vi "Dashboard Main.vi"() -> ()   [LabVIEW 2013]
uses:
  <vilib>/event_ctls.llb/eventvkey.ctl
  <vilib>/Rock Robotics/WPI/Dashboard/WPI_DashboardLogging Global.vi
  <vilib>/Utility/config.llb/Write Key (String).vi
  <vilib>/Utility/config.llb/Write Key (I32).vi
  <vilib>/Utility/config.llb/NI_LVConfig.lvlib
panel:
  out "Image Message":string="Timeout in Camera Communications"
  in  "Rec Mode":enum32{"Stop", "Record", "Playback"}(radio)
  in  "Dashboard Tab":T1(tab)
  in  "Camera Settings":T2={"Frame Rate"=30, "Compression"=30, "Size"=1} {"Frame Rate" scale=1.0..30.0; "Size" items=["640x480", "320x240", "160x120"]}
  out "MotorSliders R":T3 {"MotorSlide2 2" scale=-1.0..1.0 scale format="%#_2e"; "MotorSlide2" scale=-1.0..1.0 scale format="%#_2e"; "MotorSlide1" scale=-1.0..1.0 scale format="%#_2e"}
  out "MotorSliders L":T4 {"MotorSlide2" scale=-1.0..1.0 scale format="%#_2e"; "MotorSlide2 2" scale=-1.0..1.0 scale format="%#_2e"; "MotorSlide4 2" scale=0.0..14.0 scale format="%#_2e"; "MotorSlide1" scale=-1.0..1.0 scale format="%#_2e"}
  out "MotorChart L":T5(graph)
  out "JS1 Z":dbl(slide) scale=-1.0..1.0 scale format="%#_2e"
  out "L Joystick":cluster{"X":dbl, "Y":dbl}[](graph)
  out "JS Buttons 1":T6
  out "JS2 Z":dbl(slide) scale=-1.0..1.0 scale format="%#_2e"
  out "R Joystick":cluster{"X":dbl, "Y":dbl}[](graph)
  out "JS Buttons 2":T6
  out "Mode":T7(ring)=enum."Auto Disabled"
  out "Camera IP":string
  in  "DB Camera Config":bool
  out "fps":dbl format="%#.1g"
  out "Mbps":dbl format="%#.1g"
  out "Mbps 2":bool
  out "Target Cnt (RPi)":dbl
  out "Target Cnt (RIO)":dbl
  out "MotorChart R":T8(graph)
  in  "Enable Vision":bool
  in  "Slider 1":dbl(slide) scale=0.0..100.0
  in  "Checkbox 2":bool
  in  "Checkbox 1":bool
  in  "Test Slider":dbl(slide) scale=0.0..100.0 scale format="%#_3g"
  in  "On/Off":bool caption="Solenoid"
  in  "Test Name":u16(ring) items=["Select the test to run...", "Example Test", "-------------------------------", "List of tests is built in robot code.", "Replace with your own automated tests."]
  in  "Test Tree":string(tree)
  in  "Motor":cluster{"Value":dbl, "Enable":bool} {"Value" scale=-1.0..1.0 scale format="%#_3g"}
  out "Progress":T9 {"Test Progress" scale=0.0..100.0}
  in  "Rev/Fwd":cluster{"Forward":bool, "Reverse":bool}
  in  "Test Ring":u16(ring) items=["Auto", "Fixed indoor", "Fixed outdoor 1", "Fixed outdoor 2", "Fixed fluorescent 1", "Fixed fluorescent 2", "Hold current"]
  in  "Listbox":i32(listbox)
  out "Tree":string(tree)
  out "Camera Image":T10(plugin-control)
  in  "Enable":bool
  # "Left"
  # "Front"
  # "Right"
  # "Battery"
  # "Customize by placing controls and indicators here and name to\nmatch Dashboard Variables on robot."
  # "This tab is a great place for autonomous settings and validation.\nCustomize by placing controls and indicators here and name to\nmatch Dashboard Variables on robot."
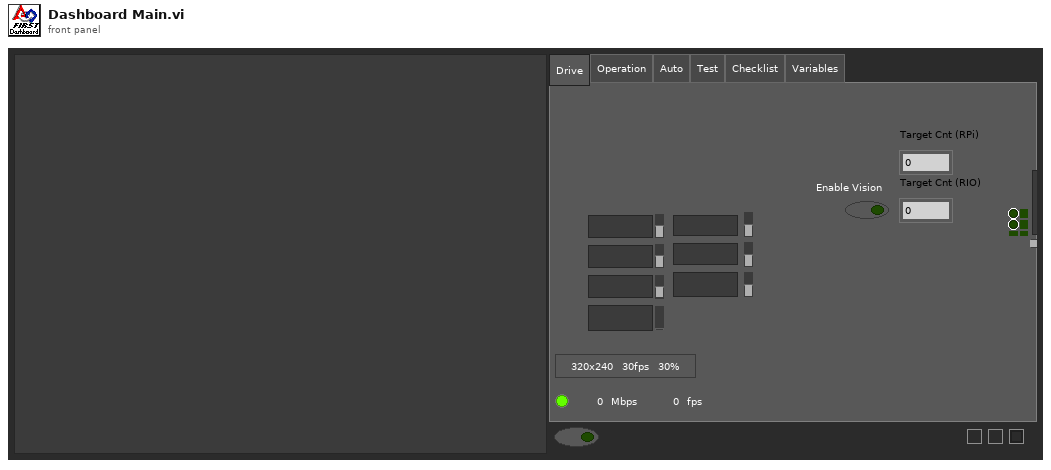
[diagram p1: front panel]
types:
  T1 = enum32{"Drive", "Operation", "Auto", "Test", "Checklist", "Variables"}
  T2 = cluster{"Frame Rate":i32, "Compression":i32, "Size":u16}
  T3 = cluster{"MotorSlide1":dbl, "MotorSlide2":dbl, "MotorSlide2 2":dbl}
  T4 = cluster{"MotorSlide1":dbl, "MotorSlide4 2":dbl, "MotorSlide2 2":dbl, "MotorSlide2":dbl}
  T5 = cluster{"Numeric":dbl, "Numeric":dbl, "Numeric":dbl, "Battery":sgl}
  T6 = cluster{bool, bool, bool, bool, bool, bool, bool, bool, bool, bool, bool, bool}
  T7 = enum8{"Tele-Op Disabled", "Tele-Op Enabled", "Auto Disabled", "Auto Enabled", "Test Disabled", "Test Enabled", ""}
  T8 = cluster{"Numeric":dbl, "Numeric":dbl, "Numeric":dbl}
  T9 = cluster{"Test Progress":u8, "Test Progress Text":string}
  T10 = typedef "IMAQ Image.ctl" = refnum<image>
  T11 = typedef "Image Type" = u32
  T12 = cluster{"Digital Inputs":bool[], "Digital Outputs":bool[]}
  T13 = cluster{"Competition mode":bool, "Robot Link":bool, "Autonomous":bool, "Enabled":bool, "E-Stop":bool, "Simulated":bool, "TestMode":bool, "Docked Window":bool}
  T14 = cluster{"Boolean Array[0]":bool, "Boolean Array[1]":bool, "Boolean Array[2]":bool, "Boolean Array[3]":bool, "Boolean Array[4]":bool, "Boolean Array[5]":bool, "Boolean Array[6]":bool, "Boolean Array[7]":bool, "Boolean Array[8]":bool, "Boolean Array[9]":bool, "Boolean Array[10]":bool, "Boolean Array[11]":bool}
  T15 = typedef "NI_LVConfig.lvlib/Config Data RefNum.ctl" = refnum<k1>
  T16 = typedef "eventvkey.ctl" = enum16{"ASCII", "Enter", "Return", "Shift", "Ctrl", "Alt", "Cmd", "Opt", "Caps", "NumLock", "Clear", "Break", "Up", "Down", "Left", "Right", "Insert", "Delete", "Home", "End", "PageUp", "PageDown", "Escape", "Help", "Pause", "ScrollLock", "F1", "F2", "F3", "F4", "F5", "F6", "F7", "F8", "F9", "F10", "F11", "F12", "F13", "F14", "F15", "F16", "F17", "F18", "F19", "F20", "F21", "F22", "F23", "F24", "Play", "VolumeUp", "VolumeDown", "Mute", "Two Byte Char"}
  T17 = cluster{"Image Size":bool, "Image Type":bool, "Pixel Value":bool, "ROI Information":bool, "Zoom Factor":bool}
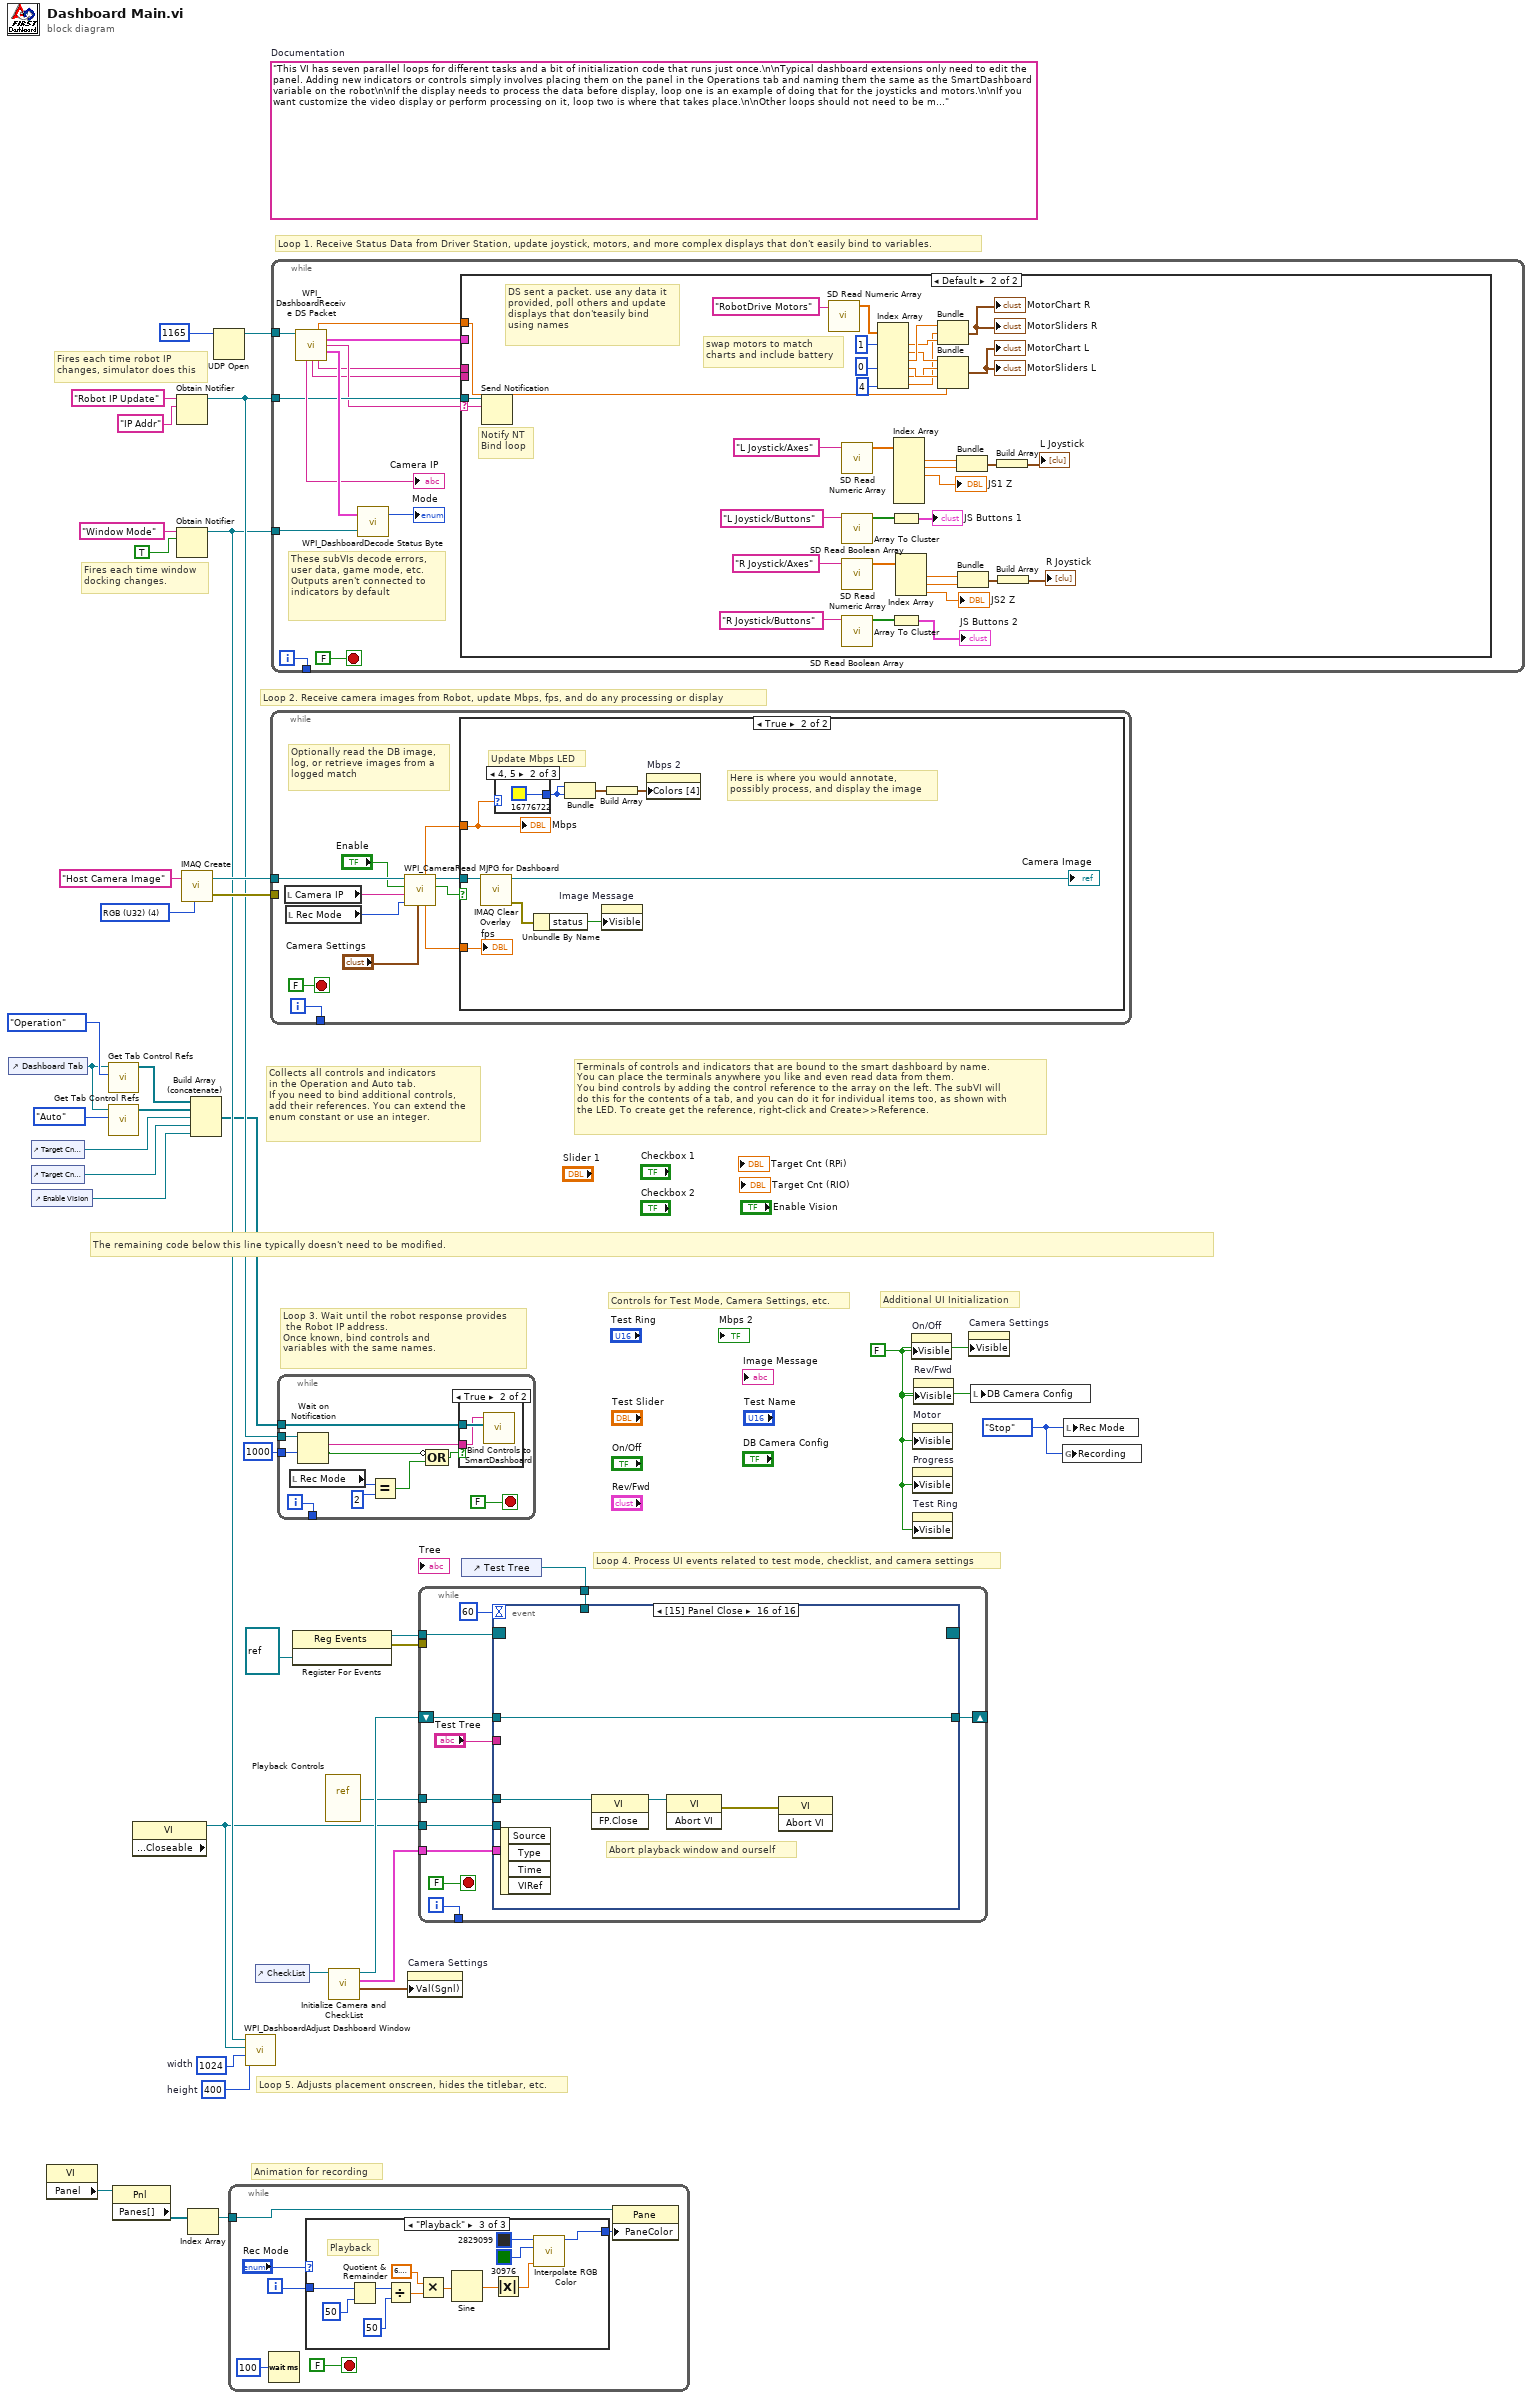
[diagram p0: block diagram]
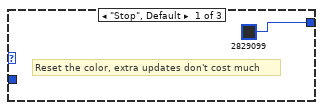
[diagram p2: hidden frame]
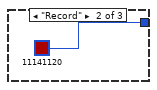
[diagram p3: hidden frame]
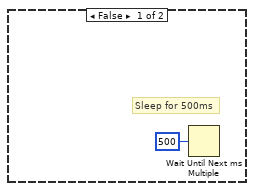
[diagram p5: hidden frame]
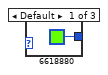
[diagram p6: hidden frame]
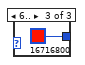
[diagram p7: hidden frame]
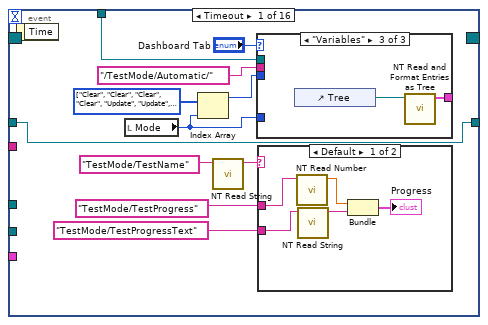
[diagram p8: hidden frame]
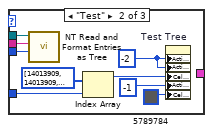
[diagram p10: hidden frame]
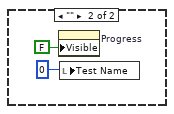
[diagram p11: hidden frame]
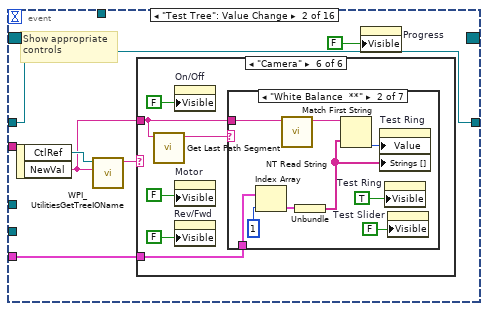
[diagram p12: hidden frame]
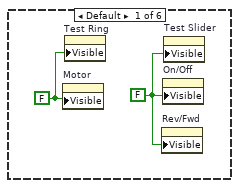
[diagram p13: hidden frame]
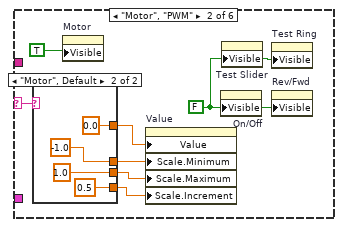
[diagram p14: hidden frame]
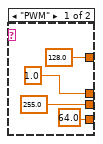
[diagram p15: hidden frame]
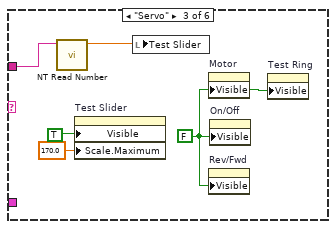
[diagram p16: hidden frame]
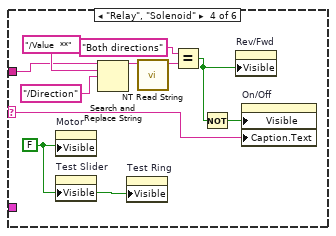
[diagram p17: hidden frame]
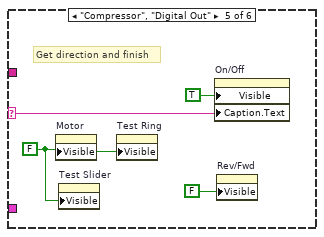
[diagram p18: hidden frame]
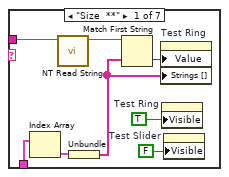
[diagram p19: hidden frame]
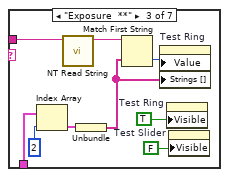
[diagram p20: hidden frame]
diagram:
  w10 = enum32{"Stop", "Record", "Playback"}."Stop" ("Rec Mode")
  w13 = 400  # height
  w14 = 1024  # width
  w27 = FALSE ("Visible")
  (unwired) "This VI has seven parallel loops for different tasks and a bit of initialization code that runs just once.\n\nTypical dashboard extensions only need to edit the panel. Adding new indicators or controls simply involves placing them on the panel in the Operations tab and naming them the same as the SmartDashboard variable on the robot\n\nIf the display needs to process the data before display, loop one is an example of doing that for the joysticks and motors.\n\nIf you want customize the video display or perform processing on it, loop two is where that takes place.\n\nOther loops should not need to be modified. They are pretty standard, and document the task they perform."  # Documentation
  w37 = T11 4 items=["Grayscale (U8)", "Grayscale (I16)", "Grayscale (SGL)", "Complex (CSG)", "RGB (U32)", "HSL (U32)", "RGB (U64)"] ("Image Type")
  # "Controls for Test Mode, Camera Settings, etc."
  # "Additional UI Initialization"
  # "Animation for recording"
  # "Fires each time robot IP\nchanges, simulator does this"
  # "Fires each time window\ndocking changes."
  # "Collects all controls and indicators\nin the Operation and Auto tab.\nIf you need to bind additional controls,\nadd their references. You can extend the\nenum constant or use an integer."
  # "The remaining code below this line typically doesn't need to be modified."
  # "Loop 4. Process UI events related to test mode, checklist, and camera settings"
  # "Terminals of controls and indicators that are bound to the smart dashboard by name.\nYou can place the terminals anywhere you like and even read data from them.\nYou bind controls by adding the control reference to the array on the left. The subVI will\ndo this for the contents of a tab, and you can do it for individual items too, as shown with\nthe LED. To create get the reference, right-click and Create>>Reference."
  # "Loop 3. Wait until the robot response provides\n the Robot IP address.\nOnce known, bind controls and\nvariables with the same names."
  # "Loop 5. Adjusts placement onscreen, hides the titlebar, etc."
  # "Loop 1. Receive Status Data from Driver Station, update joystick, motors, and more complex displays that don't easily bind to variables."
  # "Loop 2. Receive camera images from Robot, update Mbps, fps, and do any processing or display"
  n1 = control-ref of="Dashboard Tab"() -> (w8:refnum<vi>)
  n2 = control-ref of="Target Cnt (RPi)"() -> (w3:refnum<vi>)
  n3 = control-ref of="Target Cnt (RIO)"() -> (w2:refnum<vi>)
  n4 = control-ref of="Enable Vision"() -> (w1:refnum<vi>)
  n5 = property class="VI"() -> ("Panel"=w21:refnum<vi>)  [unwired: 2 in, 2 out]
  n6 = call <vilib>:"Get Tab Control Refs.vi"("Page Index"=T1."Operation" ("Dashboard Tab"), "TabControl in"=w8) -> ("ControlsOnPage"=w6:refnum<vi>[])  [unwired: 9 in]
  n7 = call <vilib>:"Get Tab Control Refs.vi"("Page Index"=T1."Auto" ("Dashboard Tab"), "TabControl in"=w8) -> ("ControlsOnPage"=w7:refnum<vi>[])  [unwired: 9 in]
  n8 = property class="Pnl"(reference=w21) -> ("Panes[]"=w22:refnum<vi>[])  [unwired: 1 in, 2 out]
  n9 = property class="VI" props=["Front Panel.Closeable"]() -> (reference out=w9:refnum<vi>)  [unwired: 2 in, 2 out]
  n10 = Obtain Notifier(name (unnamed)="Robot IP Update", notification data type="IP Addr" ("name (unnamed)")) -> (notifier out=w31:refnum<notifier>)  [unwired: 2 in, 2 out]
  n11 = Obtain Notifier(name (unnamed)="Window Mode", notification data type=TRUE) -> (notifier out=w12:refnum<notifier>)  [unwired: 2 in, 2 out]
  n12 = call "IMAQ Create"("Image Name"="Host Camera Image", "Image Type"=w37) -> ("New Image"=w35:T10, "error out"=w34:errorcluster)  [unwired: 2 in, 1 out]
  n13 = Index Array(array=w22) -> (element=w20:refnum<vi>)  [unwired: 1 in]
  n14 = Build Array (concatenate)(w6, w7, w3, w2, w1) -> (w5:refnum<vi>[])
  n15 = UDP Open(11:u16 1165 ("port")) -> (port=w38:refnum<k16>)  [unwired: 2 in, 4 out]
  n16 = while {
    tunnel: w20 -> [w41]
    i -> [w44]
    stop <- FALSE stop-if-true
    n17 = Wait (ms)(milliseconds to wait=u32 100) -> ()  [unwired: 1 out]
    n18 = case shown="\"Playback\"" "Rec Mode" {
      tunnel: w44 -> [_ _ w59]
      tunnel: [u32 2829099 ("Base Color") u32 11141120 ("Target Color") w48] -> w40
      frame "Stop", Default {
        # "Reset the color, extra updates don't cost much"
      }
      frame "Record" {
      }
      frame "Playback" {
        # "Playback"
        n19 = Quotient & Remainder(x=w59, y=u32 50 ("milliseconds to wait")) -> (x-y*floor(x/y)=w55:u32)  [unwired: 1 out]
        n20 = Divide(x=w55, y=u32 50 ("milliseconds to wait")) -> (x/y=w52:dbl)
        n21 = Multiply(x=6.283185307179586, y=w52) -> (x*y=w57:dbl)
        n22 = Sine(x=w57) -> (sin(x)=w56:dbl)
        n23 = Absolute Value(x=w56) -> (abs(x)=w49:dbl)
        n24 = call "Interpolate RGB Color.vi"("Proportion"=w49, "Target Color"=u32 30976, "Base Color"=u32 2829099) -> ("Result Color"=w48:u32)  [unwired: 8 in]
      }
    }
    n25 = property class="Pane"(reference=w41, "PaneColor"=w40) -> ()  [unwired: 1 in, 2 out]
  }
  n26 = call <vilib>:"WPI_DashboardAdjust Dashboard Window.vi"("height"=w13, "width"=w14, "reference in"=w9, "Notifier in"=w12) -> ()  [unwired: 8 in]
  n27 = control-ref of="CheckList"() -> (w11:refnum<vi>)
  n28 = while {
    tunnel: w35 -> [w68]
    tunnel: w34 -> [_]
    tunnel: [w69] -> _
    i -> [w69]
    stop <- FALSE stop-if-true
    # "Optionally read the DB image,\nlog, or retrieve images from a\nlogged match"
    n29 = local read "Camera IP"() -> (w61:string)
    n30 = local read "Rec Mode"() -> (w60:enum32{"Stop", "Record", "Playback"})
    n31 = call <vilib>:"WPI_CameraRead MJPG for Dashboard.vi"("Camera Settings"="Camera Settings", "Rec Mode"=w60, "Camera IP"=w61, "Enable"="Enable", "Refnum in"=w68) -> ("Active"=w65:bool, "Refnum out"=w67:T10, "FPS"=w64:dbl, "Bandwidth (Mbps)"=w63:dbl)  [unwired: 3 in]
    n32 = case shown="True" w65 {
      tunnel: w67 -> [_ w75]
      tunnel: w63 -> [_ w74]
      tunnel: w64 -> [_ w72]
      frame False {
        # "Sleep for 500ms"
        n33 = Wait Until Next ms Multiple(millisecond multiple=u32 500) -> ()  [unwired: 1 out]
      }
      frame True {
        # "Here is where you would annotate,\npossibly process, and display the image"
        # "Update Mbps LED"
        n34 = call "IMAQ Clear Overlay"("Image"=w75) -> ("error out"=w79:errorcluster, "Image Out"=→"Camera Image":T10)  [unwired: 2 in, 7 out]
        n35 = case shown="4, 5" w74 {
          tunnel: [u32 6618880 ("Color Box") u32 16776722 ("Color Box") u32 16716800 ("Color Box")] -> w76
          frame Default {
          }
          frame 4, 5 {
          }
          frame 6.. {
          }
        }
        n36 = Unbundle By Name(w79) -> ("status"=w80:bool)
        n37 = Bundle("Color Box"=w76, "Color Box"=w76) -> (w78:cluster{"Color Box":u32, "Color Box":u32})  [unwired: 1 out]
        n38 = property on="Image Message" class="Str"("Visible"=w80) -> ()  [unwired: 2 in, 2 out]
        n39 = Build Array(w78) -> (w77:cluster{"Color Box":u32, "Color Box":u32}[])
        n40 = property on="Mbps 2" class="Bool (strict)"("Colors [4]"=w77) -> ()  [unwired: 2 in, 2 out]
        "Mbps" <- w74
        "fps" <- w72
      }
    }
  }
  n41 = while {
    tunnel: w38 -> [w94]
    tunnel: w31 -> [w89]
    tunnel: w12 -> [w93]
    tunnel: [w90] -> _
    i -> [w90]
    stop <- FALSE stop-if-true
    # "These subVIs decode errors, user data, game mode, etc.\nOutputs aren't connected to indicators by default"
    n42 = call <vilib>:"WPI_DashboardReceive DS Packet.vi"("Recv Socket"=w94) -> ("Battery"=w84:sgl, "Driver Station"=w85:T12, "Robot IP Address"=w88:string, "Status"=w95:T13, "Camera IP Address"=→"Camera IP":string, "Low Priority User Data"=w87:string, "High Priority User Data"=w86:string)  [unwired: 1 in, 7 out]
    n43 = call <vilib>:"WPI_DashboardDecode Status Byte.vi"("Window Mode Notifier"=w93, "Status"=w95) -> ("Mode"=→"Mode":T7)  [unwired: 1 out]
    n44 = case shown="Default" w88 {
      selector: w88 -> [_ w110]
      tunnel: w89 -> [_ w111]
      tunnel: w87 -> [_ _]
      tunnel: w86 -> [_ _]
      tunnel: w85 -> [_ _]
      tunnel: w84 -> [_ w104]
      frame "0.0.0.0" {
        # "DS not sending packets, or no robot exists yet.\nDon't poll the variables"
      }
      frame Default {
        # "Notify NT\nBind loop"
        # "DS sent a packet. use any data it\nprovided, poll others and update\ndisplays that don'teasily bind\nusing names"
        # "swap motors to match\ncharts and include battery"
        n45 = Send Notification(notification=w110, notifier=w111) -> ()  [unwired: 1 in, 2 out]
        n46 = call <vilib>:"SD Read Numeric Array.vi"("Name"="RobotDrive Motors") -> ("Numeric Array"=w109:dbl[])  [unwired: 8 in, 2 out]
        n47 = call <vilib>:"SD Read Numeric Array.vi"("Name"="L Joystick/Axes") -> ("Numeric Array"=w127:dbl[])  [unwired: 8 in, 2 out]
        n48 = call <vilib>:"SD Read Boolean Array.vi"("Name"="L Joystick/Buttons") -> ("Boolean Array"=w129:bool[])  [unwired: 8 in, 2 out]
        n49 = call <vilib>:"SD Read Numeric Array.vi"("Name"="R Joystick/Axes") -> ("Numeric Array"=w121:dbl[])  [unwired: 8 in, 2 out]
        n50 = call <vilib>:"SD Read Boolean Array.vi"("Name"="R Joystick/Buttons") -> ("Boolean Array"=w120:bool[])  [unwired: 8 in, 2 out]
        n51 = Index Array(array=w109, index #1=1, index #4=0, index #5=4 ("index")) -> (element #1=w100:dbl, element #2=w107:dbl, element #3=w108:dbl, element #4=w103:dbl, element #5=w101:dbl, element #6=w99:dbl)  [unwired: 3 in]
        n52 = Array To Cluster(array=w129) -> (cluster=→"JS Buttons 1":T14)
        n53 = Array To Cluster(array=w120) -> (cluster=→"JS Buttons 2":T14)
        n54 = Index Array(array=w127) -> (element #1=w124:dbl, element #2=w125:dbl, element #3=→"JS1 Z":dbl)  [unwired: 6 in, 3 out]
        n55 = Index Array(array=w121) -> (element #1=w116:dbl, element #2=w115:dbl, element #3=→"JS2 Z":dbl)  [unwired: 3 in]
        n56 = Bundle("Numeric"=w108, "Numeric"=w99, "Numeric"=w100) -> (→"MotorSliders R" →"MotorChart R":T8)  [unwired: 1 in]
        n57 = Bundle("Numeric"=w107, "Numeric"=w101, "Numeric"=w103, "Battery"=w104) -> (→"MotorChart L" →"MotorSliders L":T5)  [unwired: 1 in]
        n58 = Bundle("Numeric"=w124, "Numeric"=w125) -> (w123:cluster{"Numeric":dbl, "Numeric":dbl})  [unwired: 1 in]
        n59 = Bundle("Numeric"=w116, "Numeric"=w115) -> (w117:cluster{"Numeric":dbl, "Numeric":dbl})  [unwired: 1 in]
        n60 = Build Array(w123) -> (→"L Joystick":cluster{"Numeric":dbl, "Numeric":dbl}[])
        n61 = Build Array(w117) -> (→"R Joystick":cluster{"Numeric":dbl, "Numeric":dbl}[])
      }
    }
  }
  n62 = while {
    tunnel: w5 -> [w143]
    tunnel: w31 -> [w141]
    tunnel: [w139] -> _
    tunnel: u32 1000 ("milliseconds to wait") -> [w138]
    i -> [w139]
    stop <- FALSE stop-if-true
    n63 = local read "Rec Mode"() -> (w134:enum32{"Stop", "Record", "Playback"})
    n64 = Wait on Notification(notifier=w141, timeout in ms (-1)=w138) -> (notification=w140:string, timed out?=w136:bool)  [unwired: 2 in, 2 out]
    n65 = Equal?(x=w134, y=u16 2 ("Rec Mode")) -> (x = y?=w135:bool)
    n66 = Compound Arithmetic op=OR(invert w136, w135) -> (w137:bool)
    n67 = case shown="True" w137 {
      tunnel: w143 -> [_ w145]
      tunnel: w140 -> [_ w144]
      frame False {
      }
      frame True {
        n68 = call <vilib>:"Bind Controls to SmartDashboard.vi"("Bound Control Refs"=w145, "Server IP Address"=w144) -> ()  [unwired: 10 in]
      }
    }
  }
  n69 = register-events(refnum<vi> refnum) -> (reference out=w18:refnum<event-registration>, error out=w17:errorcluster)  [unwired: 2 in]
  n70 = vi-ref "Playback Controls.vi"() -> (w19:refnum<vi>)
  n71 = call "Initialize Camera and CheckList.vi"("ListBox in"=w11) -> ("Cluster"=w25:cluster{"value":i32, "value":i32, "index":i32}, "Array"=w26:cluster{string[]}[], "File Refnum"=w24:T15)  [unwired: 8 in]
  n72 = property on="Camera Settings" class="Clust (strict)"("Val(Sgnl)"=w25) -> ()  [unwired: 2 in, 2 out]
  n73 = control-ref of="Test Tree"() -> (w23:refnum<vi>)
  n74 = while {
    tunnel: w26 -> [w153]
    shift-right: [w152] -> _
    shift-left: w24 -> [w151]
    tunnel: [w150] -> _
    tunnel: w23 -> [w149]
    tunnel: w19 -> [w148]
    tunnel: w18 -> [w147]
    tunnel: w17 -> [_]
    tunnel: w9 -> [w146]
    i -> [w150]
    stop <- FALSE stop-if-true
    n75 = event shown="[15] Panel Close" {
      selector: w147 -> [_ _ _ _ _ _ _ _ _ _ _ _ _ _ _ _]
      dyn-events: [_ _ _ _ _ _ _ _ _ _ _ _ _ w391 _ _] -> _
      timeout: u32 60 ("milliseconds to wait") -> [_ _ _ _ _ _ _ _ _ _ _ _ _ _ _ _]
      tunnel: w149 -> [w163 _ _ _ _ _ _ _ _ _ _ _ _ _ _ _]
      tunnel: "Test Tree" -> [_ _ _ _ _ _ _ _ w360 w368 w370 w374 w382 _ _ _]
      tunnel: w153 -> [_ w187 _ _ _ _ w324 w354 _ _ _ _ _ _ _ _]
      tunnel: [w157 w186 w285 w290 w298 w310 w323 w347 w359 w366 w369 w373 w381 w393 w407 w408] -> w152
      tunnel: w151 -> [w157 w186 w285 w290 w298 w310 w322 w347 w359 w366 w369 w373 w381 w393 w407 w408]
      tunnel: w148 -> [_ _ _ _ _ _ _ _ _ _ _ _ _ w394 _ w411]
      tunnel: w146 -> [_ _ _ _ _ _ _ _ _ _ _ _ _ w389 _ _]
      event Timeout {
        w162 = enum16{"Update", "Clear"}[] [enum."Clear", enum."Clear", enum."Clear", enum."Clear", enum."Update", enum."Update", enum."Clear"] items=["Update", "Clear"]
        n76 = event-data() -> ()  [unwired: 1 in, 1 out]
        n77 = local read "Mode"() -> (w160:T7)
        n78 = Index Array(array=w162, index=w160) -> (element=w161:enum16{"Update", "Clear"})
        n79 = call <vilib>:"NT Read String.vi"("Name"="TestMode/TestName") -> ("String"=w166:string)  [unwired: 9 in, 1 out]
        n80 = case shown="\"Variables\"" "Dashboard Tab" {
          tunnel: w163 -> [_ w176 _]
          tunnel: "/TestMode/Automatic/" ("Name Pattern") -> [_ w175 _]
          tunnel: w161 -> [_ w174 _]
          tunnel: w160 -> [_ w172 _]
          tunnel: [_ _ w178] -> _
          frame "Operation", Default {
          }
          frame "Test" {
            w171 = -2 ("Active Item:Row Number")
            n81 = call <vilib>:"NT Read and Format Entries as Tree.vi"("Operation"=w174, "Name Pattern"=w175, "Tree Refnum"=w176) -> ()  [unwired: 7 in, 2 out]
            n82 = Index Array(array=u32[] [14013909, 14013909, 14013909, 14013909, 14013909, 16777215, 14013909], index=w172) -> (element=w170:u32)
            n83 = property on="Test Tree" class="Tree (strict)"("Active Item Row Number"=w171, "ActiveColNum"=w171, "CellBG"=w170, "Active Item Row Number"=-1 ("Active Item:Row Number"), "CellBG"=u32 5789784 ("Color Box")) -> ()  [unwired: 2 in, 2 out]
          }
          frame "Variables" {
            n84 = control-ref of="Tree"() -> (w177:refnum<vi>)
            n85 = call <vilib>:"NT Read and Format Entries as Tree.vi"("Tree Refnum"=w177) -> ("Formatted Strings"=w178:cluster{"Name":string, "Value":string}[])  [unwired: 9 in, 1 out]
          }
        }
        n86 = case shown="Default" w166 {
          tunnel: "TestMode/TestProgress" ("Name") -> [w180 _]
          tunnel: "TestMode/TestProgressText" ("Name") -> [w179 _]
          frame Default {
            n87 = call <vilib>:"NT Read Number.vi"("Name"=w180) -> ("Numeric"=w181:dbl)  [unwired: 9 in, 1 out]
            n88 = call <vilib>:"NT Read String.vi"("Name"=w179) -> ("String"=w182:string)  [unwired: 9 in, 1 out]
            n89 = Bundle("Numeric"=w181, "String"=w182) -> (→"Progress":cluster{"Numeric":dbl, "String":string})  [unwired: 1 in]
          }
          frame "" {
            n90 = property on="Progress" class="Clust (strict)"("Visible"=FALSE) -> ()  [unwired: 2 in, 2 out]
            n91 = local write "Test Name"(u16 0) -> ()
          }
        }
      }
      event "Test Tree": Value Change {
        # "Show appropriate\ncontrols"
        n92 = event-data() -> ("CtlRef"=w190:refnum<vi>, "NewVal"=w188:string)  [unwired: 1 in]
        n93 = call <vilib>:"WPI_UtilitiesGetTreeIOName.vi"("NewVal"=w188, "TreeControl in"=w190) -> ("I/O Name"=w191:string)  [unwired: 9 in]
        n94 = case shown="\"Camera\"" w191 {
          selector: w191 -> [_ w198 _ w216 w225 _]
          tunnel: w188 -> [_ _ w213 w215 _ w232]
          tunnel: w187 -> [_ _ _ _ _ w231]
          frame Default {
            w193 = FALSE ("Visible")
            w192 = FALSE ("Visible")
            n95 = property on="Motor" class="Clust (strict)"("Visible"=w192) -> ()  [unwired: 2 in, 2 out]
            n96 = property on="Test Ring" class="Ring (strict)"("Visible"=w192) -> ()  [unwired: 2 in, 2 out]
            n97 = property on="Rev/Fwd" class="Clust (strict)"("Visible"=w193) -> ()  [unwired: 2 in, 2 out]
            n98 = property on="On/Off" class="Bool (strict)"("Visible"=w193) -> ()  [unwired: 2 in, 2 out]
            n99 = property on="Test Slider" class="Slide (strict)"("Visible"=w193) -> ()  [unwired: 2 in, 2 out]
          }
          frame "Motor", "PWM" {
            w199 = FALSE ("Visible")
            n100 = case shown="\"Motor\", Default" w198 {
              tunnel: [1.0 ("Value") -1.0 ("Value")] -> w197
              tunnel: [255.0 ("Value") 1.0 ("Value")] -> w196
              tunnel: [128.0 ("Value") 0.0 ("Value")] -> w195
              tunnel: [64.0 ("Value") 0.5 ("Value")] -> w194
              frame "PWM" {
              }
              frame "Motor", Default {
              }
            }
            n101 = property on="Motor" class="Clust (strict)"("Visible"=TRUE) -> ()  [unwired: 2 in, 2 out]
            n102 = property on="Value" class="Slide (strict)"("Value"=w195, "Scale.Minimum"=w197, "Scale.Maximum"=w196, "Scale.Increment"=w194) -> ()  [unwired: 2 in, 2 out]
            n103 = property on="On/Off" class="Bool (strict)"("Visible"=w199) -> ()  [unwired: 2 in, 2 out]
            n104 = property on="Test Slider" class="Slide (strict)"("Visible"=w199) -> ()  [unwired: 2 in, 2 out]
            n105 = property on="Test Ring" class="Ring (strict)"("Visible"=w199) -> ()  [unwired: 2 in, 2 out]
            n106 = property on="Rev/Fwd" class="Clust (strict)"("Visible"=w199) -> ()  [unwired: 2 in, 2 out]
          }
          frame "Servo" {
            w211 = FALSE ("Visible")
            n107 = call <vilib>:"NT Read Number.vi"("Name"=w213) -> ("Numeric"=w212:dbl)  [unwired: 9 in, 1 out]
            n108 = property on="Test Slider" class="Slide (strict)"("Visible"=TRUE, "Scale.Maximum"=170.0 ("Scale.Range:Maximum")) -> ()  [unwired: 2 in, 2 out]
            n109 = local write "Test Slider"(w212) -> ()
            n110 = property on="Motor" class="Clust (strict)"("Visible"=w211) -> ()  [unwired: 2 in, 2 out]
            n111 = property on="Rev/Fwd" class="Clust (strict)"("Visible"=w211) -> ()  [unwired: 2 in, 2 out]
            n112 = property on="On/Off" class="Bool (strict)"("Visible"=w211) -> ()  [unwired: 2 in, 2 out]
            n113 = property on="Test Ring" class="Ring (strict)"("Visible"=w211) -> ()  [unwired: 2 in, 2 out]
          }
          frame "Relay", "Solenoid" {
            w214 = FALSE ("Visible")
            n114 = property on="Motor" class="Clust (strict)"("Visible"=w214) -> ()  [unwired: 2 in, 2 out]
            n115 = property on="Test Slider" class="Slide (strict)"("Visible"=w214) -> ()  [unwired: 2 in, 2 out]
            n116 = Search and Replace String(input string=w215, search string="/Value  **", replace string="/Direction") -> (result string=w221:string)  [unwired: 5 in, 3 out]
            n117 = property on="Test Ring" class="Ring (strict)"("Visible"=w214) -> ()  [unwired: 2 in, 2 out]
            n118 = call <vilib>:"NT Read String.vi"("Name"=w221) -> ("String"=w219:string)  [unwired: 9 in, 1 out]
            n119 = Equal?(x="Both directions", y=w219) -> (x = y?=w217:bool)
            n120 = Not(x=w217) -> (.not. x?=w218:bool)
            n121 = property on="Rev/Fwd" class="Clust (strict)"("Visible"=w217) -> ()  [unwired: 2 in, 2 out]
            n122 = property on="On/Off" class="Bool (strict)"("Visible"=w218, "Caption.Text"=w216) -> ()  [unwired: 2 in, 2 out]
          }
          frame "Compressor", "Digital Out" {
            w224 = FALSE ("Visible")
            # "Get direction and finish"
            n123 = property on="Motor" class="Clust (strict)"("Visible"=w224) -> ()  [unwired: 2 in, 2 out]
            n124 = property on="Test Slider" class="Slide (strict)"("Visible"=w224) -> ()  [unwired: 2 in, 2 out]
            n125 = property on="Test Ring" class="Ring (strict)"("Visible"=w224) -> ()  [unwired: 2 in, 2 out]
            n126 = property on="On/Off" class="Bool (strict)"("Visible"=TRUE, "Caption.Text"=w225) -> ()  [unwired: 2 in, 2 out]
            n127 = property on="Rev/Fwd" class="Clust (strict)"("Visible"=FALSE) -> ()  [unwired: 2 in, 2 out]
          }
          frame "Camera" {
            n128 = call <vilib>:"Get Last Path Segment.vi"("String in"=w232) -> ("String out"=w233:string)  [unwired: 10 in]
            n129 = property on="On/Off" class="Bool (strict)"("Visible"=FALSE) -> ()  [unwired: 2 in, 2 out]
            n130 = property on="Motor" class="Clust (strict)"("Visible"=FALSE) -> ()  [unwired: 2 in, 2 out]
            n131 = property on="Rev/Fwd" class="Clust (strict)"("Visible"=FALSE) -> ()  [unwired: 2 in, 2 out]
            n132 = case shown="\"White Balance  **\"" w233 {
              tunnel: w232 -> [w239 w248 w257 w266 w275 _ w281]
              tunnel: w231 -> [w237 w245 w254 w263 w272 _ _]
              frame "Size  **" {
                n133 = Index Array(array=w237) -> (element=w236:cluster{string[]})  [unwired: 1 in]
                n134 = call <vilib>:"NT Read String.vi"("Name"=w239) -> ("String"=w238:string)  [unwired: 9 in, 1 out]
                n135 = Unbundle(w236) -> (w234:string[])
                n136 = Match First String(2:w234, 3:w238) -> (0:w235:i32)  [unwired: 1 out]
                n137 = property on="Test Ring" class="Ring (strict)"("Value"=w235, "Strings []"=w234) -> ()  [unwired: 2 in, 2 out]
                n138 = property on="Test Ring" class="Ring (strict)"("Visible"=TRUE) -> ()  [unwired: 2 in, 2 out]
                n139 = property on="Test Slider" class="Slide (strict)"("Visible"=FALSE) -> ()  [unwired: 2 in, 2 out]
              }
              frame "White Balance  **" {
                n140 = Index Array(array=w245, index=1) -> (element=w246:cluster{string[]})
                n141 = call <vilib>:"NT Read String.vi"("Name"=w248) -> ("String"=w247:string)  [unwired: 9 in, 1 out]
                n142 = Unbundle(w246) -> (w243:string[])
                n143 = Match First String(2:w243, 3:w247) -> (0:w242:i32)  [unwired: 1 out]
                n144 = property on="Test Ring" class="Ring (strict)"("Value"=w242, "Strings []"=w243) -> ()  [unwired: 2 in, 2 out]
                n145 = property on="Test Ring" class="Ring (strict)"("Visible"=TRUE) -> ()  [unwired: 2 in, 2 out]
                n146 = property on="Test Slider" class="Slide (strict)"("Visible"=FALSE) -> ()  [unwired: 2 in, 2 out]
              }
              frame "Exposure  **" {
                n147 = Index Array(array=w254, index=2) -> (element=w255:cluster{string[]})
                n148 = call <vilib>:"NT Read String.vi"("Name"=w257) -> ("String"=w256:string)  [unwired: 9 in, 1 out]
                n149 = Unbundle(w255) -> (w251:string[])
                n150 = Match First String(2:w251, 3:w256) -> (0:w252:i32)  [unwired: 1 out]
                n151 = property on="Test Ring" class="Ring (strict)"("Value"=w252, "Strings []"=w251) -> ()  [unwired: 2 in, 2 out]
                n152 = property on="Test Ring" class="Ring (strict)"("Visible"=TRUE) -> ()  [unwired: 2 in, 2 out]
                n153 = property on="Test Slider" class="Slide (strict)"("Visible"=FALSE) -> ()  [unwired: 2 in, 2 out]
              }
              frame "Exposure Priority  **" {
                n154 = Index Array(array=w263, index=3) -> (element=w264:cluster{string[]})
                n155 = call <vilib>:"NT Read String.vi"("Name"=w266) -> ("String"=w265:string)  [unwired: 9 in, 1 out]
                n156 = Unbundle(w264) -> (w260:string[])
                n157 = Match First String(2:w260, 3:w265) -> (0:w261:i32)  [unwired: 1 out]
                n158 = property on="Test Ring" class="Ring (strict)"("Value"=w261, "Strings []"=w260) -> ()  [unwired: 2 in, 2 out]
                n159 = property on="Test Ring" class="Ring (strict)"("Visible"=TRUE) -> ()  [unwired: 2 in, 2 out]
                n160 = property on="Test Slider" class="Slide (strict)"("Visible"=FALSE) -> ()  [unwired: 2 in, 2 out]
              }
              frame "Color Enable  **" {
                n161 = Index Array(array=w272, index=4) -> (element=w273:cluster{string[]})
                n162 = call <vilib>:"NT Read String.vi"("Name"=w275) -> ("String"=w274:string)  [unwired: 9 in, 1 out]
                n163 = Unbundle(w273) -> (w269:string[])
                n164 = Match First String(2:w269, 3:w274) -> (0:w270:i32)  [unwired: 1 out]
                n165 = property on="Test Ring" class="Ring (strict)"("Value"=w270, "Strings []"=w269) -> ()  [unwired: 2 in, 2 out]
                n166 = property on="Test Ring" class="Ring (strict)"("Visible"=TRUE) -> ()  [unwired: 2 in, 2 out]
                n167 = property on="Test Slider" class="Slide (strict)"("Visible"=FALSE) -> ()  [unwired: 2 in, 2 out]
              }
              frame Default {
                n168 = property on="Test Ring" class="Ring (strict)"("Visible"=FALSE) -> ()  [unwired: 2 in, 2 out]
                n169 = property on="Test Slider" class="Slide (strict)"("Visible"=FALSE) -> ()  [unwired: 2 in, 2 out]
              }
              frame "Brightness  **", "Color Level  **", "Compression  **", "FPS  **", "Sharpness  **" {
                n170 = call <vilib>:"NT Read Number.vi"("Name"=w281) -> ("Numeric"=w280:dbl)  [unwired: 9 in, 1 out]
                n171 = local write "Test Slider"(w280) -> ()
                n172 = property on="Test Slider" class="Slide (strict)"("Visible"=TRUE, "Scale.Maximum"=100.0 ("Scale.Range:Maximum")) -> ()  [unwired: 2 in, 2 out]
                n173 = property on="Test Ring" class="Ring (strict)"("Visible"=FALSE) -> ()  [unwired: 2 in, 2 out]
              }
            }
          }
        }
        n174 = property on="Progress" class="Clust (strict)"("Visible"=FALSE) -> ()  [unwired: 2 in, 2 out]
      }
      event "Test Name": Mouse Enter {
        # "Populate the ring with the list of tests"
        n175 = event-data() -> ()  [unwired: 1 in, 1 out]
        n176 = call <vilib>:"NT Read String Array.vi"("Name"="TestMode/TestList") -> ("String Array"=w289:string[])  [unwired: 9 in, 1 out]
        n177 = Build Array (concatenate)("Select the test to run...", w289) -> (w288:string[])
        n178 = property on="Test Name" class="Ring (strict)"("Strings []"=w288) -> ()  [unwired: 2 in, 2 out]
      }
      event "Test Name": Value Change {
        w291 = FALSE ("Visible")
        # "Tell the robot the test name to run"
        n179 = event-data() -> ("NewVal"=w295:u16)  [unwired: 1 in]
        n180 = property on="Test Name" class="Ring (strict)"() -> ("Strings []"=w296:string[])  [unwired: 2 in, 2 out]
        n181 = local write "Progress"(T9 {"Test Progress"=0, "Test Progress Text"=""} ("Progress")) -> ()
        n182 = Index Array(array=w296, index=w295) -> (element=w294:string)
        n183 = call <vilib>:"NT Write String.vi"("String"=w294, "Name"="TestMode/TestName") -> ()  [unwired: 9 in, 1 out]
        n184 = property on="Progress" class="Clust (strict)"("Visible"=TRUE) -> ()  [unwired: 2 in, 2 out]
        n185 = property on="Motor" class="Clust (strict)"("Visible"=w291) -> ()  [unwired: 2 in, 2 out]
        n186 = property on="Test Slider" class="Slide (strict)"("Visible"=w291) -> ()  [unwired: 2 in, 2 out]
        n187 = property on="On/Off" class="Bool (strict)"("Visible"=w291) -> ()  [unwired: 2 in, 2 out]
        n188 = property on="Rev/Fwd" class="Clust (strict)"("Visible"=w291) -> ()  [unwired: 2 in, 2 out]
        n189 = property on="Test Ring" class="Ring (strict)"("Visible"=w291) -> ()  [unwired: 2 in, 2 out]
      }
      event "Listbox": Double Click {
        n190 = event-data() -> ("PlatMods.Shift"=w299:bool, "Row"=w301:i32)  [unwired: 1 in]
        n191 = case shown="True" w299 {
          tunnel: w301 -> [w305 _]
          tunnel: 1 -> [w304 _]
          frame False {
            n192 = property on="Listbox" class="LstBox (strict)"() -> ("Item Symbols"=w303:i32[])  [unwired: 2 in, 2 out]
            n193 = Replace Array Subset(array=w303, new element=w304, index=w305) -> (w302:i32[])
            n194 = property on="Listbox" class="LstBox (strict)"("Item Symbols"=w302) -> ()  [unwired: 2 in, 2 out]
          }
          frame True {
            w306 = 0 ("Top Row")
            n195 = property on="Listbox" class="LstBox (strict)"() -> ("Number of Rows"=w308:u32)  [unwired: 2 in, 2 out]
            n196 = Initialize Array(0, w308) -> (w307:i32[])
            n197 = property on="Listbox" class="LstBox (strict)"("Top Row"=w306, "Value"=w306, "Item Symbols"=w307) -> ()  [unwired: 2 in, 2 out]
          }
        }
      }
      event "Listbox": Key Down {
        n198 = event-data() -> ("VKey"=w312:T16)  [unwired: 1 in]
        n199 = case shown="\"Left\", \"Right\"" w312 {
          selector: w312 -> [w317 _]
          tunnel: eventvkey."Left" ("VKey") -> [w315 _]
          frame "Left", "Right" {
            n200 = Equal?(x=w315, y=w317) -> (x = y?=w316:bool)
            n201 = Select(t=0, s=w316, f=1) -> (s? t:f=w318:i32)
            n202 = property on="Listbox" class="LstBox (strict)"() -> ("Item Symbols"=w321:i32[])  [unwired: 2 in, 2 out]
            n203 = Replace Array Subset(array=w321, new element=w318, index="Listbox") -> (w320:i32[])
            n204 = property on="Listbox" class="LstBox (strict)"("Item Symbols"=w320) -> ()  [unwired: 2 in, 2 out]
          }
          frame Default {
          }
        }
      }
      event "DB Camera Config": Value Change {
        n205 = event-data() -> ("NewVal"=w325:bool)  [unwired: 1 in]
        n206 = case shown="False" w325 {
          tunnel: w324 -> [w334 _]
          tunnel: [w327 w345] -> w323
          tunnel: w322 -> [w326 w345]
          frame False {
            w341 = "Camera"
            w344 = FALSE ("Visible")
            n207 = local read "Camera Settings"() -> (w333:T2)
            n208 = Index Array(array=w334) -> (element=w337:cluster{string[]})  [unwired: 1 in]
            n209 = Unbundle(w333) -> ("Frame Rate"=w332:i32, "Compression"=w331:i32, "Size"=w335:u16)
            n210 = Unbundle(w337) -> (w336:string[])
            n211 = Index Array(array=w336, index=w335) -> (element=w330:string)
            n212 = call-poly <vilib>:"Write Key.vi"("section"=w341, "value"=w330, "key"="Size", "refnum"=w326) -> ("refnum out"=w343:T15)  [unwired: 2 in, 5 out]
            n213 = call-poly <vilib>:"Write Key.vi"("section"=w341, "value"=w332, "key"="FrameRate", "refnum"=w343) -> ("refnum out"=w342:T15)  [unwired: 1 in, 6 out]
            n214 = property on="Camera Settings" class="Clust (strict)"("Visible"=w344) -> ()  [unwired: 2 in, 2 out]
            n215 = local write "DB Camera Config"(w344) -> ()
            n216 = call-poly <vilib>:"Write Key.vi"("section"=w341, "value"=w331, "key"="Compression", "refnum"=w342) -> ("refnum out"=w328:T15)  [unwired: 1 in, 6 out]
            n217 = call <vilib>:"Close Config Data.vi"("refnum"=w328) -> ("file path"=w329:path)  [unwired: 2 in, 8 out]
            n218 = call <vilib>:"Open Config Data.vi"("configuration file path"=w329) -> ("refnum"=w327:T15)  [unwired: 8 in, 2 out]
          }
          frame True {
            n219 = property on="Camera Settings" class="Clust (strict)"("Visible"=TRUE) -> ()  [unwired: 2 in, 2 out]
          }
        }
      }
      event "Camera Settings": Value Change {
        n220 = event-data() -> ("NewVal"=w358:T2)  [unwired: 1 in]
        n221 = Index Array(array=w354) -> (element=w353:cluster{string[]})  [unwired: 1 in]
        n222 = Unbundle(w358) -> ("Frame Rate"=w349:i32, "Compression"=w348:i32, "Size"=w351:u16)
        n223 = Unbundle(w353) -> (w352:string[])
        n224 = Index Array(array=w352, index=w351) -> (element=w350:string)
        n225 = Format Into String(format string="%s   %dfps   %d%%", w350, w349, w348) -> (resulting string=w355:string)  [unwired: 2 in, 1 out]
        n226 = Build Array(w355) -> (w356:string[])
        n227 = property on="DB Camera Config" class="Bool (strict)"("Strings [4]"=w356) -> ()  [unwired: 2 in, 2 out]
      }
      event "Motor.Enable": Value Change {
        n228 = event-data() -> ("NewVal"=w364:bool)  [unwired: 1 in]
        n229 = Unbundle("Motor") -> ("Value"=w363:dbl)  [unwired: 1 out]
        n230 = Select(t=w363, s=w364, f=0.0) -> (s? t:f=w361:dbl)
        n231 = call <vilib>:"NT Write Number.vi"("Numeric"=w361, "Name"=w360) -> ()  [unwired: 9 in, 1 out]
      }
      event "Test Slider": Value Change {
        n232 = event-data() -> ("NewVal"=w367:dbl)  [unwired: 1 in]
        n233 = call <vilib>:"NT Write Number.vi"("Numeric"=w367, "Name"=w368) -> ()  [unwired: 9 in, 1 out]
      }
      event "On/Off": Value Change {
        n234 = event-data() -> ("NewVal"=w372:bool)  [unwired: 1 in]
        n235 = Boolean To (0,1)(Boolean=w372) -> (0, 1=w371:i16)
        n236 = call <vilib>:"NT Write Number.vi"("Numeric"=w371, "Name"=w370) -> ()  [unwired: 9 in, 1 out]
      }
      event "Rev/Fwd": Value Change {
        n237 = event-data() -> ("NewVal.Forward"=w380:bool, "NewVal.Reverse"=w379:bool)  [unwired: 1 in]
        n238 = Boolean To (0,1)(Boolean=w380) -> (0, 1=w376:i16)
        n239 = Boolean To (0,1)(Boolean=w379) -> (0, 1=w378:i16)
        n240 = Negate(x=w378) -> (-x=w377:i16)
        n241 = Add(x=w376, y=w377) -> (x+y=w375:i16)
        n242 = call <vilib>:"NT Write Number.vi"("Numeric"=w375, "Name"=w374) -> ()  [unwired: 9 in, 1 out]
      }
      event "Test Ring": Value Change {
        n243 = event-data() -> ("NewVal"=w384:u16)  [unwired: 1 in]
        n244 = property on="Test Ring" class="Ring (strict)"() -> ("Strings []"=w385:string[])  [unwired: 2 in, 2 out]
        n245 = Index Array(array=w385, index=w384) -> (element=w383:string)
        n246 = call <vilib>:"NT Write String.vi"("String"=w383, "Name"=w382) -> ()  [unwired: 9 in, 1 out]
      }
      event "Rec Mode": Value Change {
        # "Update globals for recording mode and path to read log from.\nClear when logging and let NetworkTables set path for vision to\nuse."
        n247 = event-data() -> ("NewVal"=w395:enum32{"Stop", "Record", "Playback"})  [unwired: 1 in]
        n248 = global write "WPI_DashboardLogging Global.vi" "Logging Filename"(path "") -> ()
        n249 = case shown="\"Stop\", \"Record\"" w395 {
          tunnel: w394 -> [_ w397 w405]
          tunnel: [_ _ w404] -> w391
          tunnel: [_ _ w403] -> _
          tunnel: w389 -> [_ _ w401]
          tunnel: cluster{i32, i32} {-250, 170} -> [_ _ w400]
          tunnel: [_ _ T17 {"Image Size"=TRUE, "Image Type"=TRUE, "Pixel Value"=TRUE, "ROI Information"=TRUE, "Zoom Factor"=FALSE} ("Image Information Shown:All Elements")] -> w387
          tunnel: [_ _ TRUE ("Zoom Factor")] -> w386
          frame Default {
          }
          frame "Stop", "Record" {
            # "Place Window too"
            n250 = invoke class="VI" method="FP.Close"(reference=w397) -> (reference out=w396:refnum<vi>)  [unwired: 2 in, 2 out]
            n251 = invoke class="VI" method="Abort VI"(reference=w396) -> ()  [unwired: 2 in, 3 out]
          }
          frame "Playback" {
            n252 = call "Open Playback Panel.vi"("Offset"=w400, "DB VI Ref"=w401, "Playback in"=w405) -> ("Playback out"=w402:refnum<vi>)  [unwired: 8 in]
            n253 = register-events(w402) -> (reference out=w404:refnum<event-registration>, error out=w403:errorcluster)  [unwired: 2 in]
          }
        }
        n254 = global write "WPI_DashboardLogging Global.vi" "Recording"(w395) -> ()
        n255 = property on="Camera Image" class="ImageControl"("Image Information Shown"=w387, "Image Information Visible"=w386) -> ()  [unwired: 2 in, 2 out]
        n256 = call <vilib>:"WPI_DashboardNT Log FieldName Cache.vi"("Operation"=enum16{"Lookup/Add", "Index", "Clear"}."Clear") -> ()  [unwired: 8 in, 3 out]
      }
      event Panel Close {
        w406 = enum32{"Stop", "Record", "Playback"}."Stop" ("Rec Mode")
        n257 = event-data() -> ()  [unwired: 1 in, 4 out]
        n258 = local write "Rec Mode"(w406) -> ()
        n259 = global write "WPI_DashboardLogging Global.vi" "Recording"(w406) -> ()
      }
      event Panel Close {
        # "Abort playback window and ourself"
        n260 = event-data() -> ()  [unwired: 1 in, 4 out]
        n261 = invoke class="VI" method="FP.Close"(reference=w411) -> (reference out=w410:refnum<vi>)  [unwired: 2 in, 2 out]
        n262 = invoke class="VI" method="Abort VI"(reference=w410) -> (error out=w409:errorcluster)  [unwired: 2 in, 2 out]
        n263 = invoke class="VI" method="Abort VI"(error in=w409) -> ()  [unwired: 2 in, 3 out]
      }
    }
  }
  n264 = property on="On/Off" class="Bool (strict)"("Visible"=w27) -> ()  [unwired: 2 in, 2 out]
  n265 = property on="Motor" class="Clust (strict)"("Visible"=w27) -> ()  [unwired: 2 in, 2 out]
  n266 = property on="Progress" class="Clust (strict)"("Visible"=w27) -> ()  [unwired: 2 in, 2 out]
  n267 = property on="Test Ring" class="Ring (strict)"("Visible"=w27) -> ()  [unwired: 2 in, 2 out]
  n268 = property on="Rev/Fwd" class="Clust (strict)"("Visible"=w27) -> ()  [unwired: 2 in, 2 out]
  n269 = property on="Camera Settings" class="Clust (strict)"("Visible"=w27) -> ()  [unwired: 2 in, 2 out]
  n270 = local write "DB Camera Config"(w27) -> ()
  n271 = global write "WPI_DashboardLogging Global.vi" "Recording"(w10) -> ()
  n272 = local write "Rec Mode"(w10) -> ()
